vi "Read Section.vi"(8 "error in (no error)":errorcluster caption="错误输入（无错误）", 11 "section":string caption="段") -> (0 "error out":errorcluster caption="错误输出", 2 "Value":string[](array[string]), 3 "key names":string[](array[string]) caption="键名")   [LabVIEW 2013, in "Resource Constant.lvlib"]
uses:
  Resource Constant.lvlib
  <vilib>/Utility/config.llb/Read Key (String).vi
  <vilib>/Utility/config.llb/NI_LVConfig.lvlib
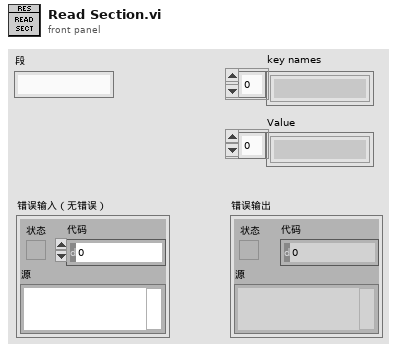
[diagram p1: front panel]
types:
  T1 = typedef "NI_LVConfig.lvlib/Config Data RefNum.ctl" = refnum<k1>
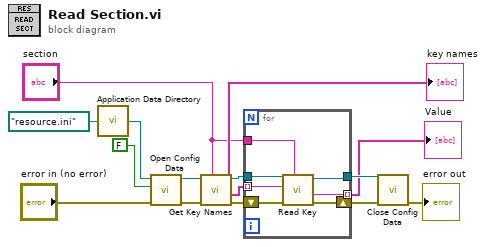
[diagram p0: block diagram]
diagram:
  n1 = call "Application Data Directory.vi"("Relative path (.)"=path "resource.ini") -> ("Application Directory (+ Relative)"=w13:path)
  n2 = call <vilib>:"Open Config Data.vi"("error in (no error)"="error in (no error)", "create file if necessary (T)"=FALSE, "configuration file path"=w13) -> ("error out"=w6:errorcluster, "refnum"=w9:T1)  [unwired: 6 in, 1 out]
  n3 = call <vilib>:"Get Key Names.vi"("section"="section", "error in (no error)"=w6, "refnum"=w9) -> ("error out"=w5:errorcluster, "key names"=w10:string[], "refnum out"=w11:T1)  [unwired: 5 in, 1 out]
  "key names" <- w10
  n4 = for {
    tunnel: w10 -> [w21] mode=indexing
    tunnel: w11 -> [w20]
    tunnel: [w19] -> w7 mode=indexing
    tunnel: [w18] -> w8
    tunnel: "section" -> [w17]
    shift-right: [w15] -> w4
    shift-left: w5 -> [w16]
    n5 = call-poly <vilib>:"Read Key.vi"("section"=w17, "error in (no error)"=w16, "key"=w21, "refnum"=w20) -> ("error out"=w15:errorcluster, "value"=w19:string, "refnum out"=w18:T1)  [unwired: 4 in, 1 out]
  }
  "Value" <- w7
  n6 = call <vilib>:"Close Config Data.vi"("error in (no error)"=w4, "refnum"=w8) -> ("error out"=→"error out":errorcluster)  [unwired: 8 in, 1 out]
